vi "Set-Exposure-mode.vi"(8 "error in (no error)":errorcluster, 10 "Acquis. params. ref. in":refnum<data-value>, 11 "Camera in":refnum<class "Camera.lvclass">) -> (0 "error out":errorcluster, 2 "Acquis. params. ref.":refnum<data-value>, 3 "Camera out":refnum<class "Camera.lvclass">)   [LabVIEW 2013, in "CameraVision.lvlib" / "Camera.lvclass"]
uses:
  Camera.lvclass
  Main/Acquisition/CV-Acquisition.lvclass
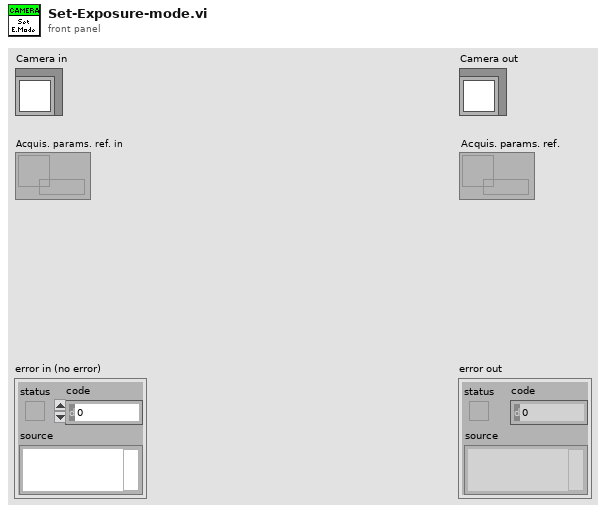
[diagram p1: front panel]
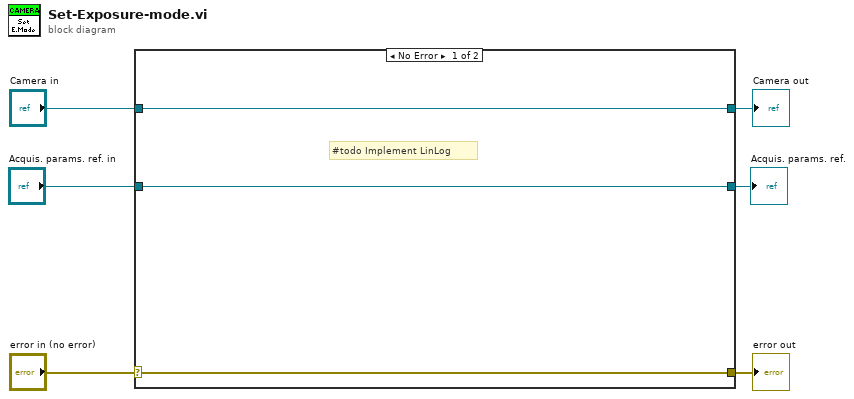
[diagram p0: block diagram]
diagram:
  n1 = case shown="No Error" "error in (no error)" {
    selector: "error in (no error)" -> [w8 w12]
    tunnel: [w8 w12] -> w5
    tunnel: [w9 w11] -> w3
    tunnel: "Camera in" -> [w9 w11]
    tunnel: "Acquis. params. ref. in" -> [w7 w10]
    tunnel: [w7 w10] -> w1
    frame No Error {
      # "#todo Implement LinLog"
    }
    frame Error {
    }
  }
  "error out" <- w5
  "Camera out" <- w3
  "Acquis. params. ref." <- w1
